vi "WaitForBusTrigger.vi"(8 "Error In":errorcluster, 10 "Timeout (sec)":dbl, 11 "Keithley 2602 In":refnum<visa-resource-name>) -> (0 "Error Out":errorcluster, 2 "Trigger Detected?":bool, 3 "Keithley 2602 Out":refnum<visa-resource-name>)   [LabVIEW 2013, in "Keithley-2602.lvlib"]
uses:
  Keithley-2602.lvlib
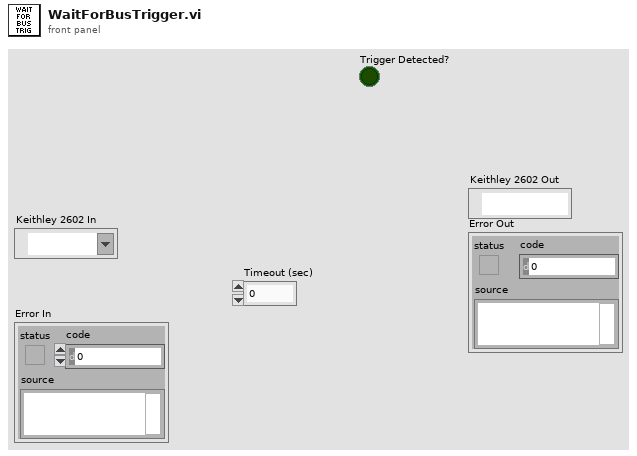
[diagram p1: front panel]
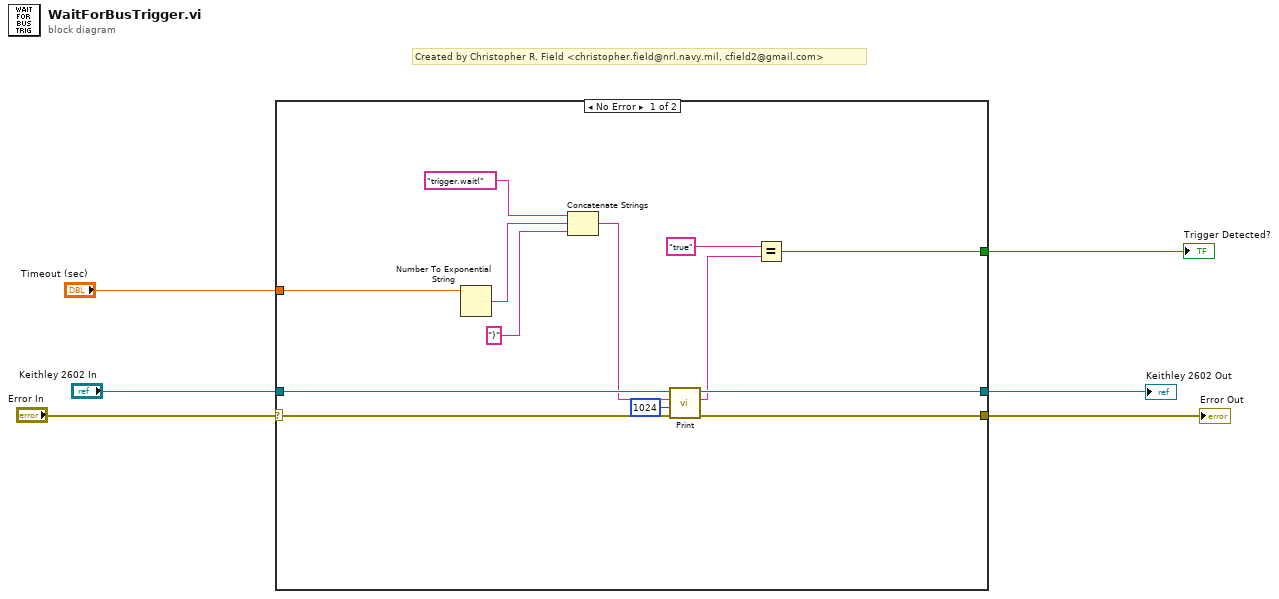
[diagram p0: block diagram]
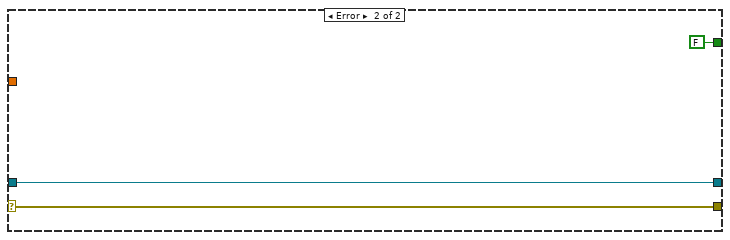
[diagram p2: hidden frame]
diagram:
  # "Created by Christopher R. Field <christopher.field@nrl.navy.mil, cfield2@gmail.com>"
  n1 = case shown="No Error" "Error In" {
    selector: "Error In" -> [w9 w21]
    tunnel: "Timeout (sec)" -> [w18 _]
    tunnel: "Keithley 2602 In" -> [w17 w22]
    tunnel: [w15 w22] -> w4
    tunnel: [w14 w21] -> w3
    tunnel: [w10 FALSE] -> w2
    frame No Error {
      n2 = Number To Exponential String(number=w18) -> (E-format string=w8:string)  [unwired: 3 in]
      n3 = Concatenate Strings("trigger.wait(", w8, ")" ("string")) -> (w16:string)
      n4 = call "Print.vi"("Error In"=w9, "Byte Count"=u32 1024, "Attribute"=w16, "Kiethley 2602 In"=w17) -> ("Error Out"=w14:errorcluster, "Output"=w12:string, "Keithley 2602 Out"=w15:refnum<visa-resource-name>)  [unwired: 5 in]
      n5 = Equal?(x="true", y=w12) -> (x = y?=w10:bool)
    }
    frame Error {
    }
  }
  "Keithley 2602 Out" <- w4
  "Error Out" <- w3
  "Trigger Detected?" <- w2
